vi "-8301 Item not found in JSON--error.vi"(8 "error in":errorcluster, 11 "$Path or Item Name":string) -> (0 "error out":errorcluster)   [LabVIEW 2025, in "Common Helpers.lvlib"]
uses:
  Common Helpers.lvlib
  Error Helpers.lvlib
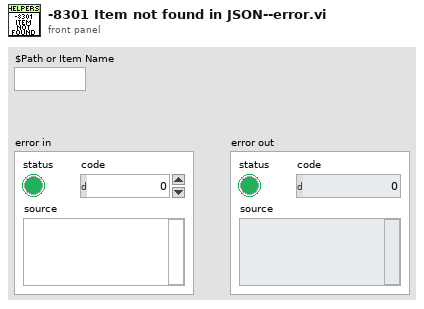
[diagram p1: front panel]
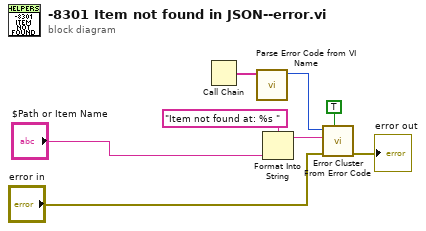
[diagram p0: block diagram]
diagram:
  n1 = Call Chain() -> (call chain=w2:string[])
  n2 = call "Parse Error Code from VI Name.vi"("Call Chain"=w2) -> ("Error Code"=w1:i32)  [unwired: 10 in]
  n3 = Format Into String(format string="Item not found at: %s " ("string"), "$Path or Item Name") -> (resulting string=w3:string)  [unwired: 2 in, 1 out]
  n4 = call <vilib>:"Error Cluster From Error Code.vi"("show call chain? (False)"=TRUE, "error in (no error)"="error in", "error message (\"\")"=w3, "error code (0)"=w1) -> ("error out"=→"error out":errorcluster)  [unwired: 5 in]
